vi "Create Menu Divider.vi"(4 "error in (no error)":errorcluster) -> (0 "error out":errorcluster, 3 "MenuItem":refnum<k24>)   [LabVIEW 2020, in "NotifyIcon.lvlib"]
uses:
  NotifyIcon.lvlib
  System.Windows.Forms
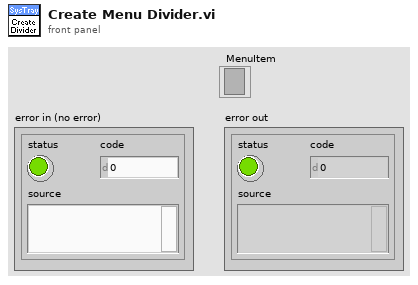
[diagram p1: front panel]
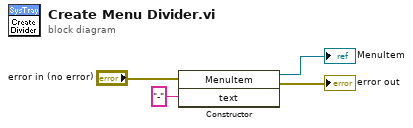
[diagram p0: block diagram]
diagram:
  n1 = constructor class="MenuItem"(error in="error in (no error)", "text"="-" ("String text")) -> (reference out=→"MenuItem":refnum<k24>, error out=→"error out":errorcluster)  [unwired: 2 in, 2 out]
